vi "Add to Queue.vi"(8 "error in (no error)":errorcluster, 9 "Front? (F)":bool, 10 "Actions":T1[](array[typedef]), 11 "Queue Ref In":refnum<queue>) -> (0 "error out":errorcluster, 3 "Queue Ref Out":refnum<queue>)   [LabVIEW 2018]
uses:
  Exec Action.ctl
  Actions.ctl
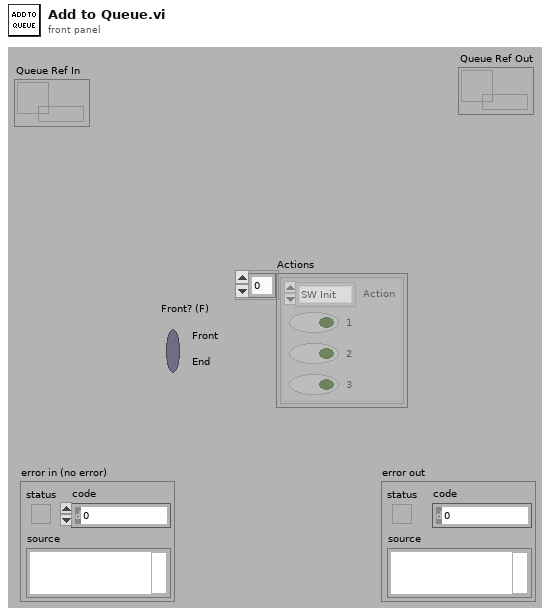
[diagram p1: front panel]
types:
  T1 = typedef "Exec Action.ctl" = cluster{"Action":T2, "1":bool, "2":bool, "3":bool}
  T2 = typedef "Actions.ctl" = enum16{"SW Init", "HW Init - Zaber", "HW Init - DO", "Init Asynch Vis", "Set Motion Params", "Set Zout Pos", "Set Zstart Pos", "Step Z", "Method close - Shear force", "Method close - SICM", "Method close - Keyence", "Method UI and HW init", "Tune Shear Force", "Plane Set Point 1", "Plane Set Point 2", "Plane Set Point 3", "Calculate Plane", "Scan UI", "Scan Ctrl", "Handle DLADS", "XY and Sensor Init", "Z Init", "MS Trig", "Line Motion", "Z Exit Ctrl", "MS Complete", "Pause Check Ctrl", "Shift Data", "Plot Profile", "Save Scan Config", "Save Profile Text File", "Wait (ms)", "Get Time", "HW Close - Zaber", "HW Close - DO", "Error", "Exit", "Shutdown Ctrl"}
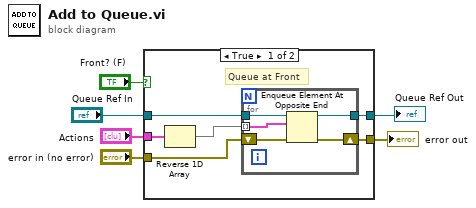
[diagram p0: block diagram]
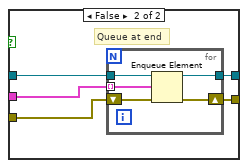
[diagram p2: hidden frame]
diagram:
  n1 = case shown="True" "Front? (F)" {
    tunnel: "Actions" -> [w12 w22]
    tunnel: [w11 w21] -> w1
    tunnel: "Queue Ref In" -> [w10 w20]
    tunnel: "error in (no error)" -> [w9 w19]
    tunnel: [w8 w18] -> w4
    frame True {
      # "Queue at Front"
      n2 = Reverse 1D Array(array=w12) -> (reversed array=w7:T1[])
      n3 = for {
        tunnel: w10 -> [w17]
        tunnel: w7 -> [w15] mode=indexing
        tunnel: [w16] -> w11
        shift-right: [w13] -> w8
        shift-left: w9 -> [w14]
        n4 = Enqueue Element At Opposite End(queue=w17, element=w15, error in (no error)=w14) -> (queue out=w16:refnum<queue>, error out=w13:errorcluster)  [unwired: 1 in, 1 out]
      }
    }
    frame False {
      # "Queue at end"
      n5 = for {
        tunnel: w20 -> [w24]
        tunnel: w22 -> [w23] mode=indexing
        tunnel: [w27] -> w21
        shift-right: [w25] -> w18
        shift-left: w19 -> [w26]
        n6 = Enqueue Element(queue=w24, element=w23, error in (no error)=w26) -> (queue out=w27:refnum<queue>, error out=w25:errorcluster)  [unwired: 1 in, 1 out]
      }
    }
  }
  "error out" <- w4
  "Queue Ref Out" <- w1
